vi "DC_CNTRL_enquire_potential.vi"(8 "error in (no error)":errorcluster, 10 "Box Number":u16(ring), 11 "Handle":u64) -> (0 "error out":errorcluster, 2 "Current Value (V)":dbl, 3 "Handle out":u64)   [LabVIEW 2019]
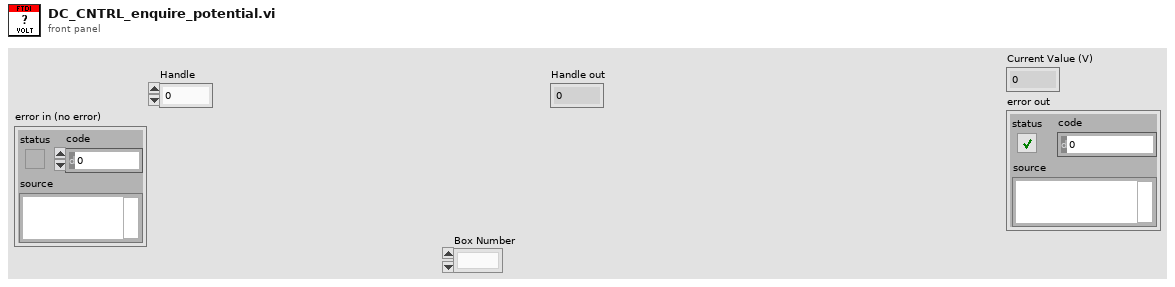
[diagram p1: front panel]
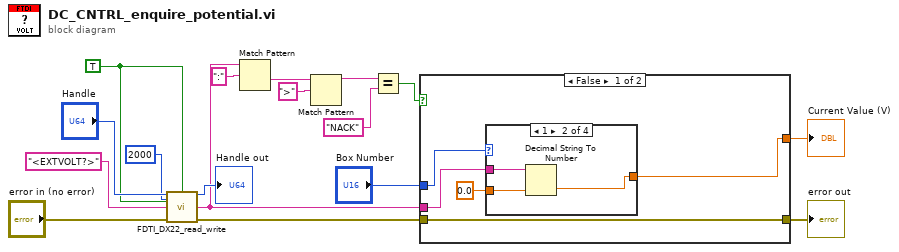
[diagram p0: block diagram]
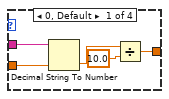
[diagram p2: hidden frame]
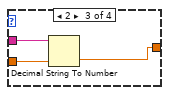
[diagram p3: hidden frame]
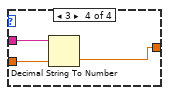
[diagram p4: hidden frame]
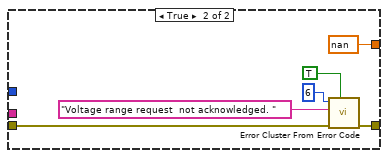
[diagram p5: hidden frame]
diagram:
  w12 = TRUE ("Clear  RxTx Buffer?")
  n1 = call "FDTI_DX22_read_write.vi"("Handle"="Handle", "Read Answer?"=w12, "Bytes wait timeout / ms"=2000, "Clear  RxTx Buffer?"=w12, "Write string"="<EXTVOLT?>" ("string"), "error in (no error)"="error in (no error)") -> ("Handle out"=→"Handle out":u64, "Read Data"=w4:string, "error out"=w5:errorcluster)  [unwired: 7 in]
  n2 = Match Pattern(string=w4, regular expression=":") -> (after substring=w10:string)  [unwired: 1 in, 3 out]
  n3 = Match Pattern(string=w10, regular expression=">") -> (before substring=w7:string)  [unwired: 1 in, 3 out]
  n4 = Equal?(x=w7, y="NACK") -> (x = y?=w8:bool)
  n5 = case shown="False" w8 {
    tunnel: w5 -> [w22 w42]
    tunnel: w4 -> [w20 _]
    tunnel: [w22 w38] -> w1
    tunnel: "Box Number" -> [w21 _]
    tunnel: [w18 nan] -> w2
    frame False {
      n6 = case shown="1" w21 {
        tunnel: w20 -> [w27 w30 w33 w36]
        tunnel: [w24 w29 w32 w35] -> w18
        tunnel: 0.0 -> [w23 w28 w31 w34]
        frame 0, Default {
          n7 = Decimal String To Number(string=w27, default (0L)=w23) -> (number=w26:dbl)  [unwired: 1 in, 1 out]
          n8 = Divide(x=w26, y=10.0) -> (x/y=w24:dbl)
        }
        frame 1 {
          n9 = Decimal String To Number(string=w30, default (0L)=w28) -> (number=w29:dbl)  [unwired: 1 in, 1 out]
        }
        frame 2 {
          n10 = Decimal String To Number(string=w33, default (0L)=w31) -> (number=w32:dbl)  [unwired: 1 in, 1 out]
        }
        frame 3 {
          n11 = Decimal String To Number(string=w36, default (0L)=w34) -> (number=w35:dbl)  [unwired: 1 in, 1 out]
        }
      }
    }
    frame True {
      n12 = call <vilib>:"Error Cluster From Error Code.vi"("show call chain? (False)"=TRUE, "error in (no error)"=w42, "error message (\"\")"="Voltage range request  not acknowledged. " ("error message (\"\")"), "error code (0)"=6) -> ("error out"=w38:errorcluster)  [unwired: 5 in]
    }
  }
  "Current Value (V)" <- w2
  "error out" <- w1
